vi "Main Page - Multi FPGA.vi"(8 "error in (no error)":errorcluster, 11 "Node Ptr":T1 format="%.0x") -> (0 "error out":errorcluster)   [LabVIEW 2015, in "Engine Simulation Toolkit System Explorer.lvlib"]
uses:
  Engine Simulation Toolkit System Explorer.lvlib
  <vilib>/NI Veristand/Custom Device API/Custom Device Item Ref.ctl
  Listbox State.ctl
  Shared/Properties.vi
  <vilib>/NI Veristand/Custom Device API/Get Item Property (I32).vi
  <vilib>/NI Veristand/Custom Device API/Get Item Property (String Array).vi
  <vilib>/NI Veristand/Custom Device API/Get Item Property (Dependent File).vi
  <vilib>/NI Veristand/Custom Device API/Get Item Property (String).vi
  <vilib>/NI Veristand/Custom Device API/Set Item Property (I32).vi
  Shared/Constants and GUIDs.vi
  <vilib>/NI Veristand/Custom Device API/Set Item Property (String Array).vi
  <vilib>/NI Veristand/Custom Device API/Set Item Property (String).vi
  <userlib>/_OpenG.lib/array/array.llb/Delete Elements from 2D Array (String)__ogtk.vi
  <vilib>/NI Veristand/Custom Device API/Custom Device API.lvlib
  Shared/Engine Simulation Toolkit Shared.lvlib
  <vilib>/NI Veristand/Custom Device Tools/Custom Device Utility Library/Custom Device Utility Library.lvlib
panel:
  in  "Reload bitfile":bool
  in  "Set master":bool
  in  "Remove bitfile":bool
  in  "Add bitfile":bool
  in  "Bitfile listbox":i32[](listbox) caption="Available APUs"
  in  "Header 3":cluster{"Section Name":string}={"Section Name"="Bitfile Selection"}
  in  "Remove APU":bool
  in  "Add APU":bool
  in  "APU listbox":i32[](listbox) caption="Available APUs"
  in  "Header 2":cluster{"Section Name":string}={"Section Name"="Available APUs"}
  in  "CPU":i32=-2
  in  "Rate decimation":i32=1 min=1
  in  "Execution priority":enum16{"Low", "Medium", "High"}(ring)=enum."Medium"
  out "CD Version":string caption="Custom device version"
  in  "Header":cluster{"Section Name":string}={"Section Name"="Engine Simulation Toolkit Settings"}
  in  "Name":string
  # "(-2: automatic)"
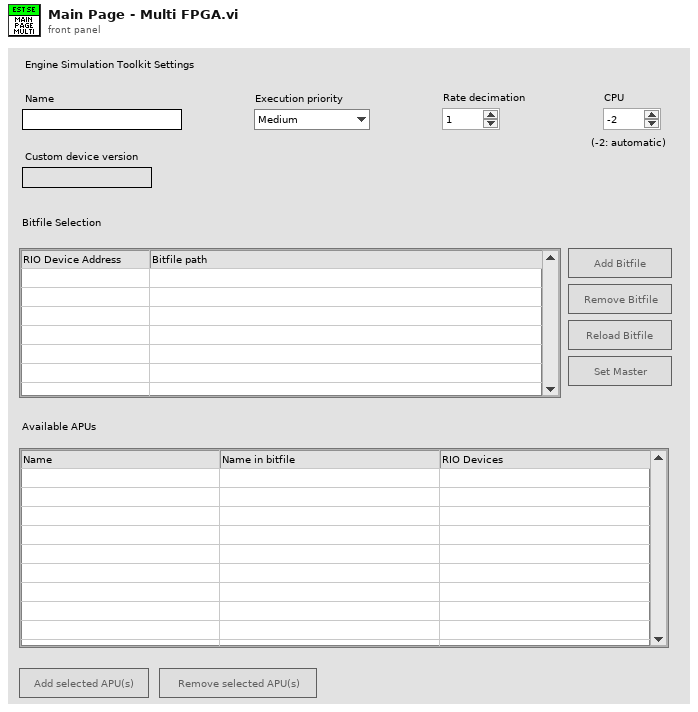
[diagram p1: front panel]
types:
  T1 = typedef "Custom Device API.lvlib/Custom Device Item Ref.ctl" = u64
  T2 = typedef "Engine Simulation Toolkit System Explorer.lvlib/Listbox State.ctl" = cluster{"listbox text":string[][], "not present item indexes":i32[], "selected values":i32[]}
  T3 = enum8{"Enabled", "Disabled", "Disabled and Grayed Out"}
  T4 = typedef "Custom Device API.lvlib/Custom Device Timed Loop Priority.ctl" = enum32{"Low", "Medium", "High"}
  T5 = typedef "Custom Device API.lvlib/Custom Device Item Info.ctl" = cluster{"Name":string, "Is Channel":bool, "GUID":string, "Is Waveform":bool}
  T6 = typedef "Custom Device API.lvlib/Custom Device Commands.ctl" = enum16{"Default", "Item renamed", "Shutdown", "Dynamic button pressed"}
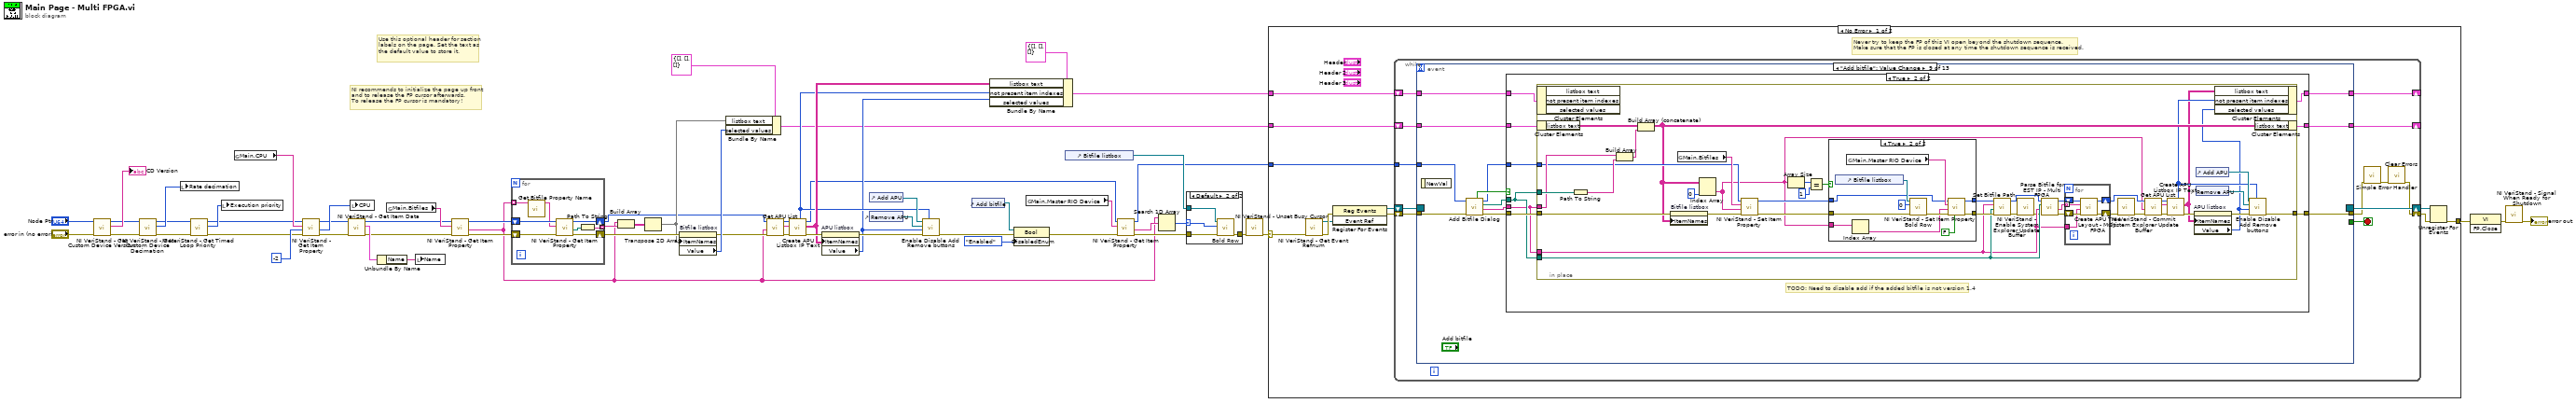
[diagram p0: block diagram]
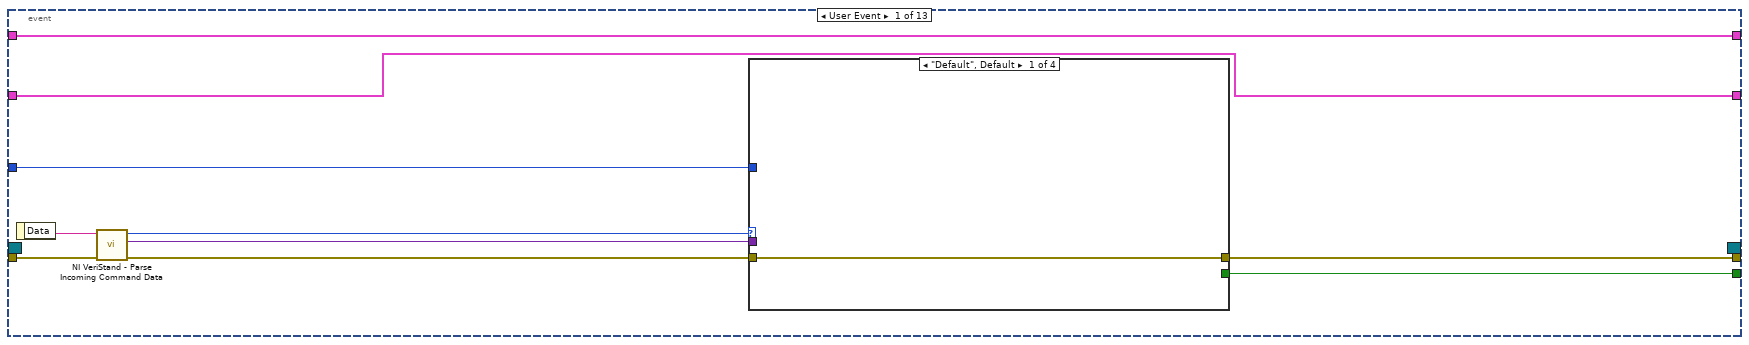
[diagram p3: hidden frame]
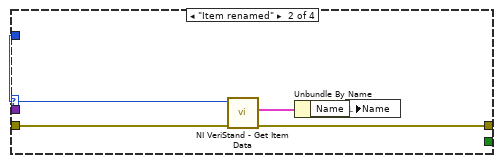
[diagram p4: hidden frame]
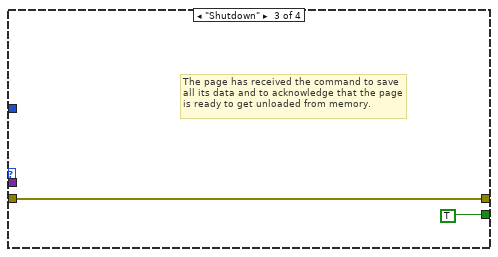
[diagram p5: hidden frame]
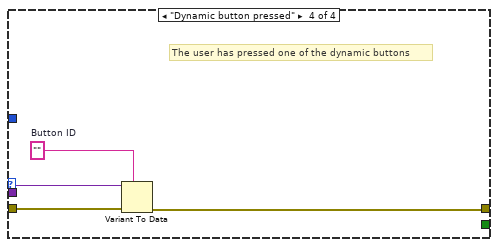
[diagram p6: hidden frame]
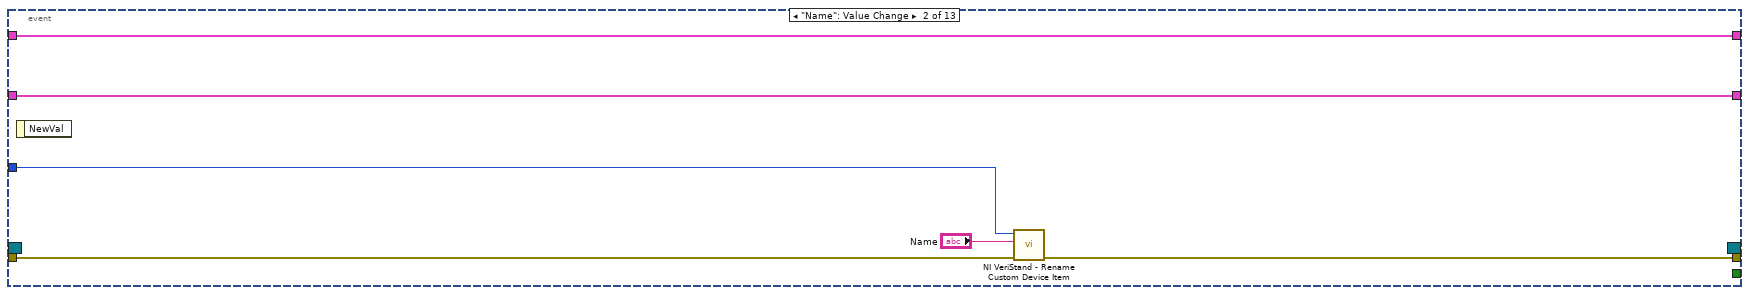
[diagram p7: hidden frame]
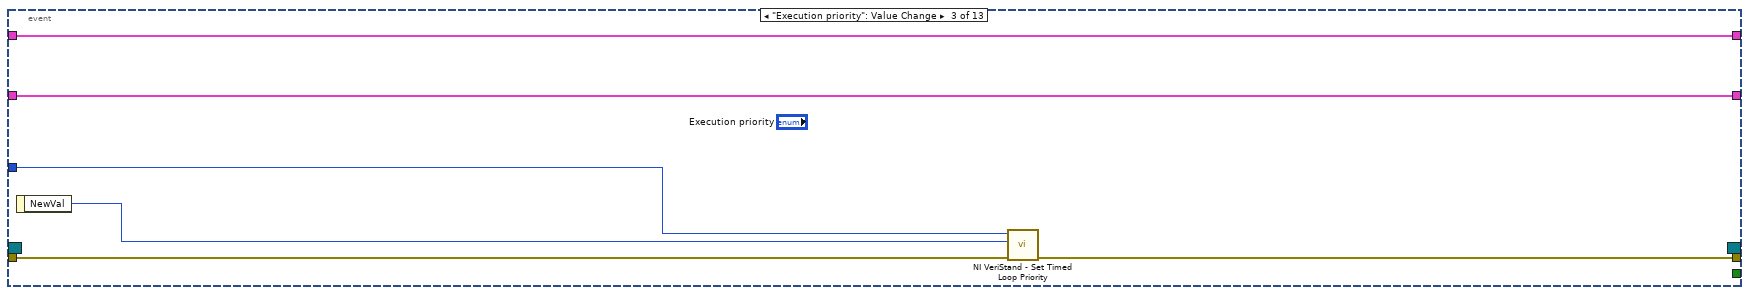
[diagram p8: hidden frame]
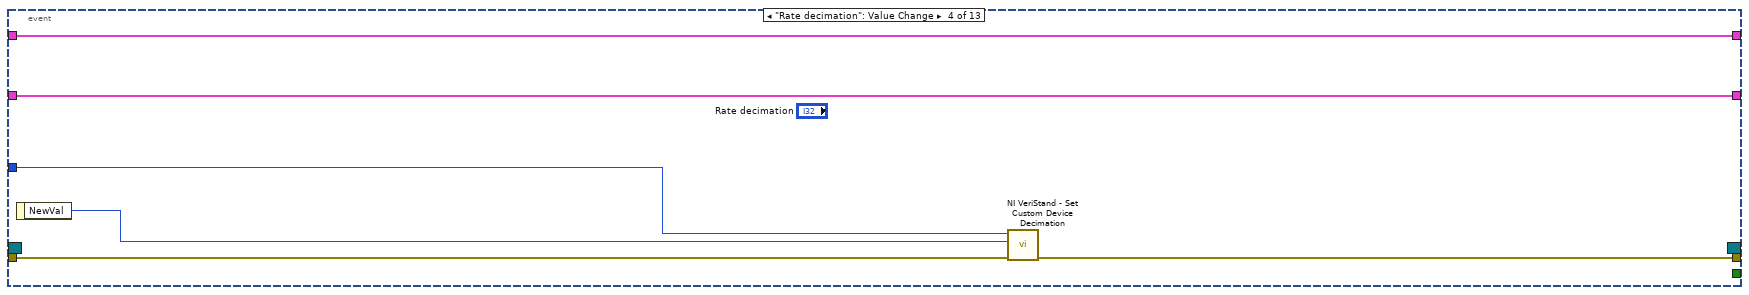
[diagram p9: hidden frame]
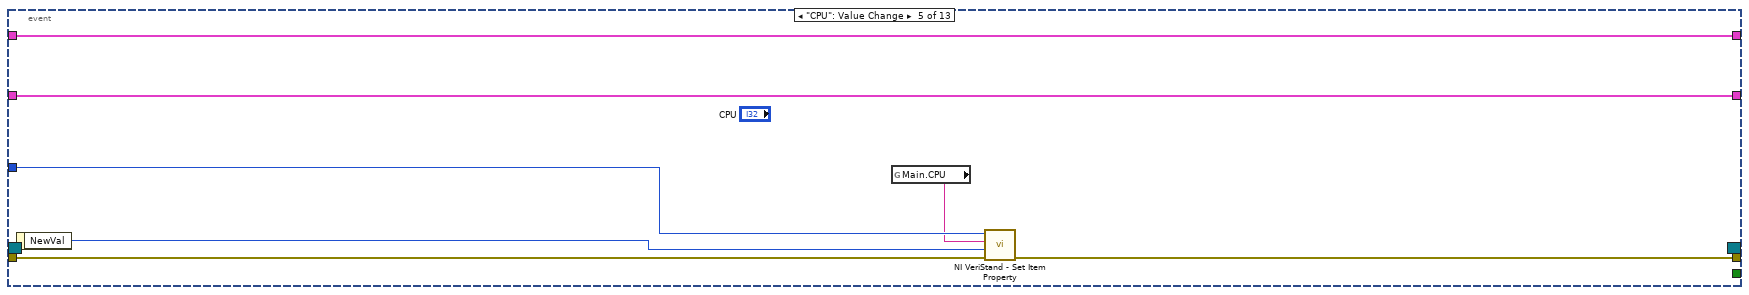
[diagram p10: hidden frame]
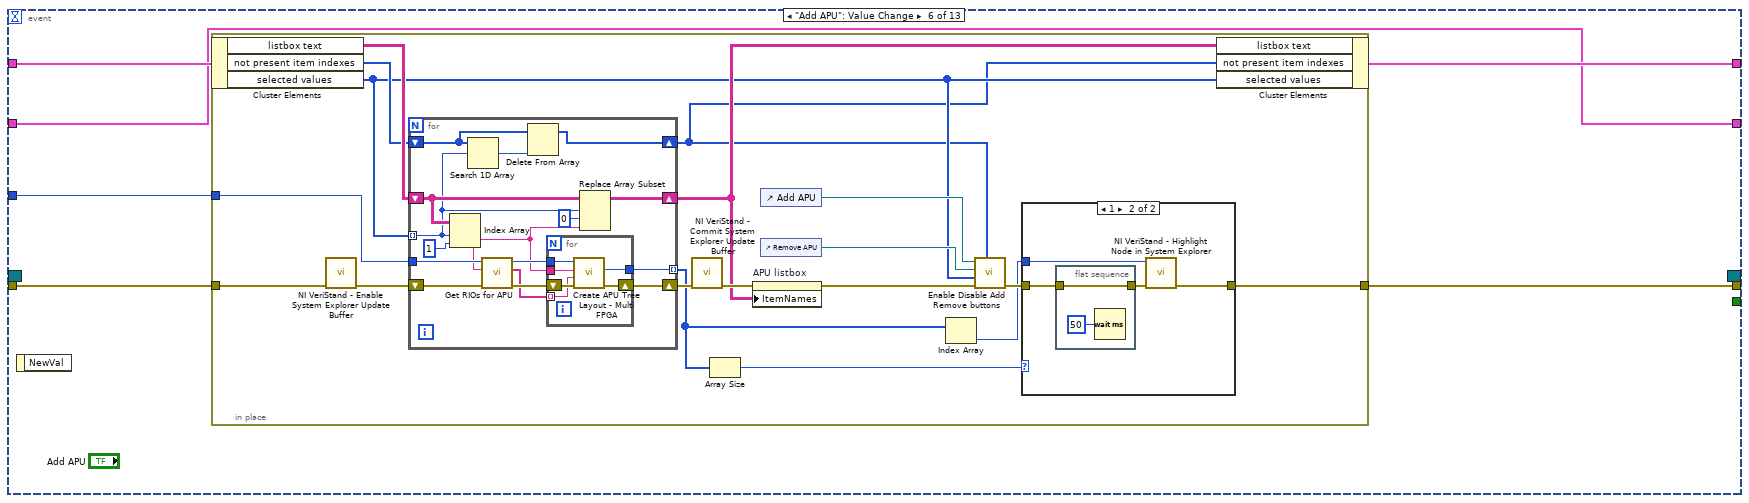
[diagram p11: hidden frame]
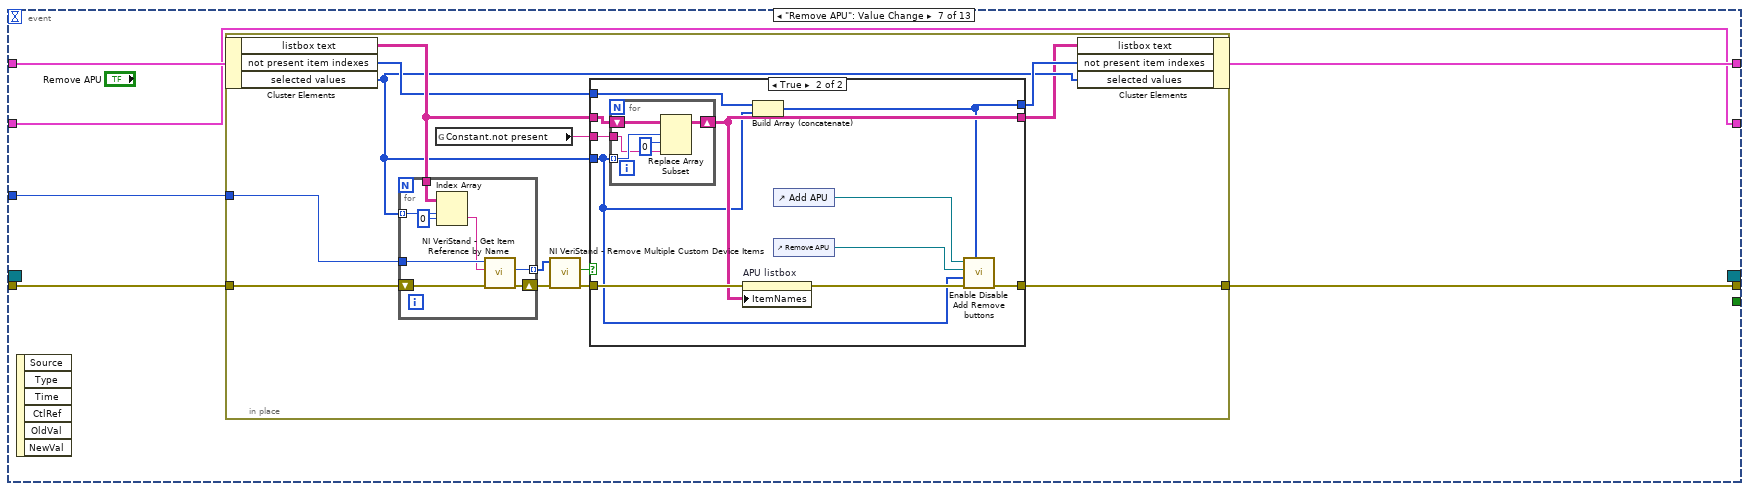
[diagram p13: hidden frame]
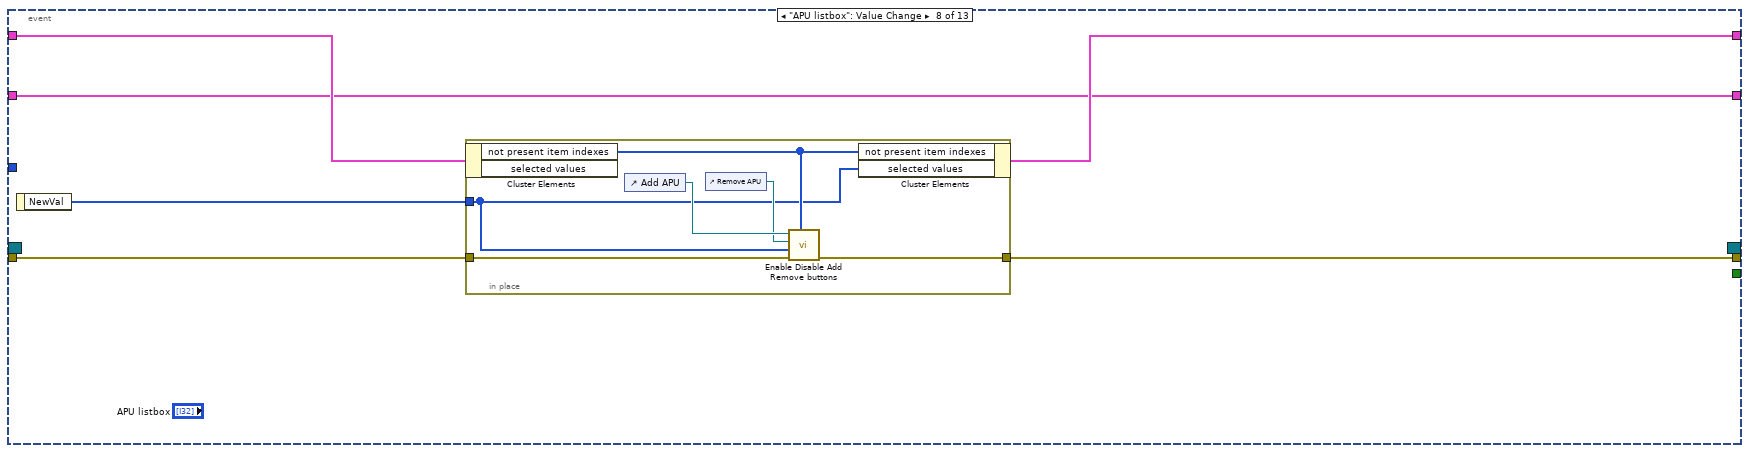
[diagram p15: hidden frame]
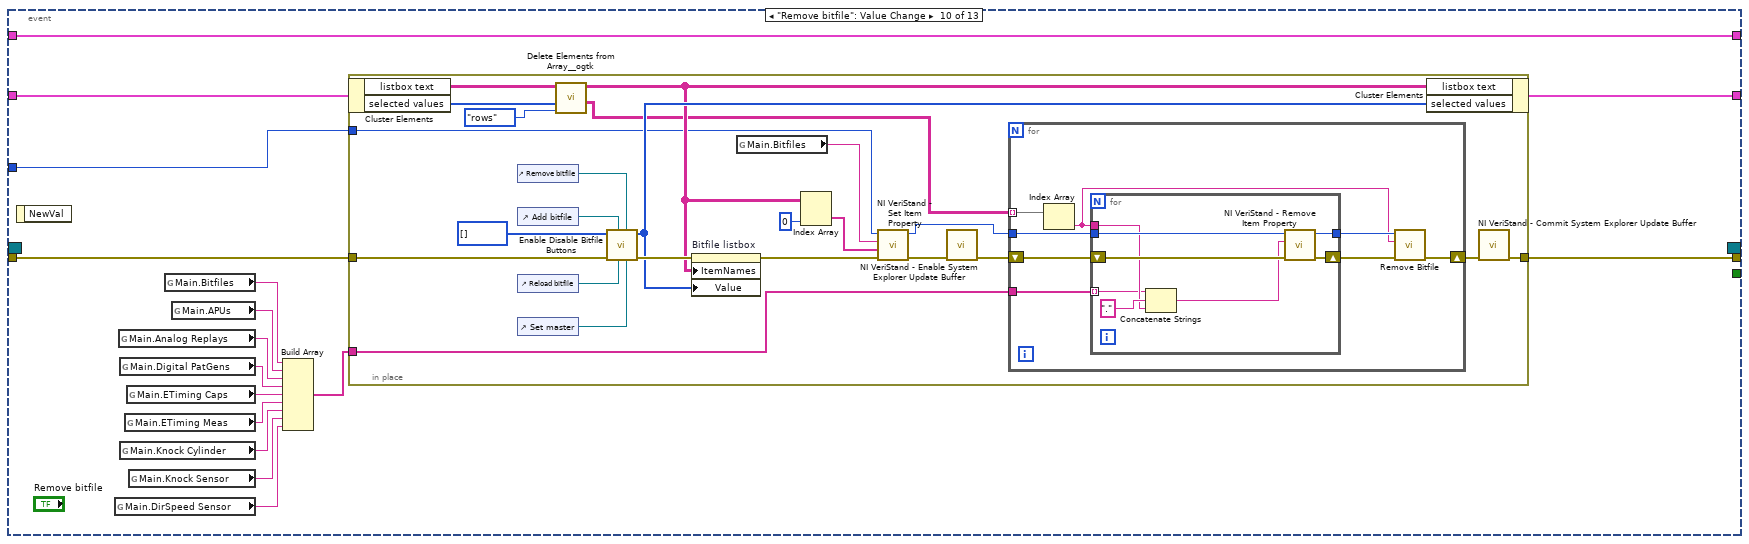
[diagram p18: hidden frame]
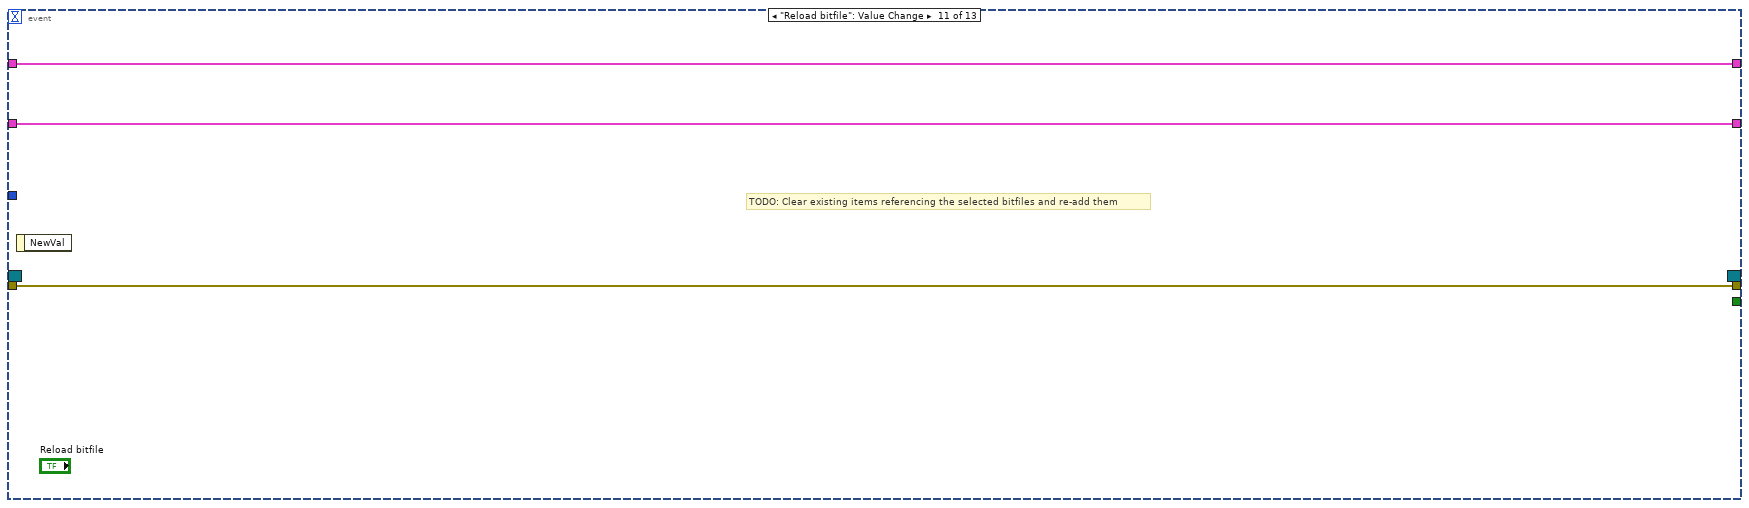
[diagram p19: hidden frame]
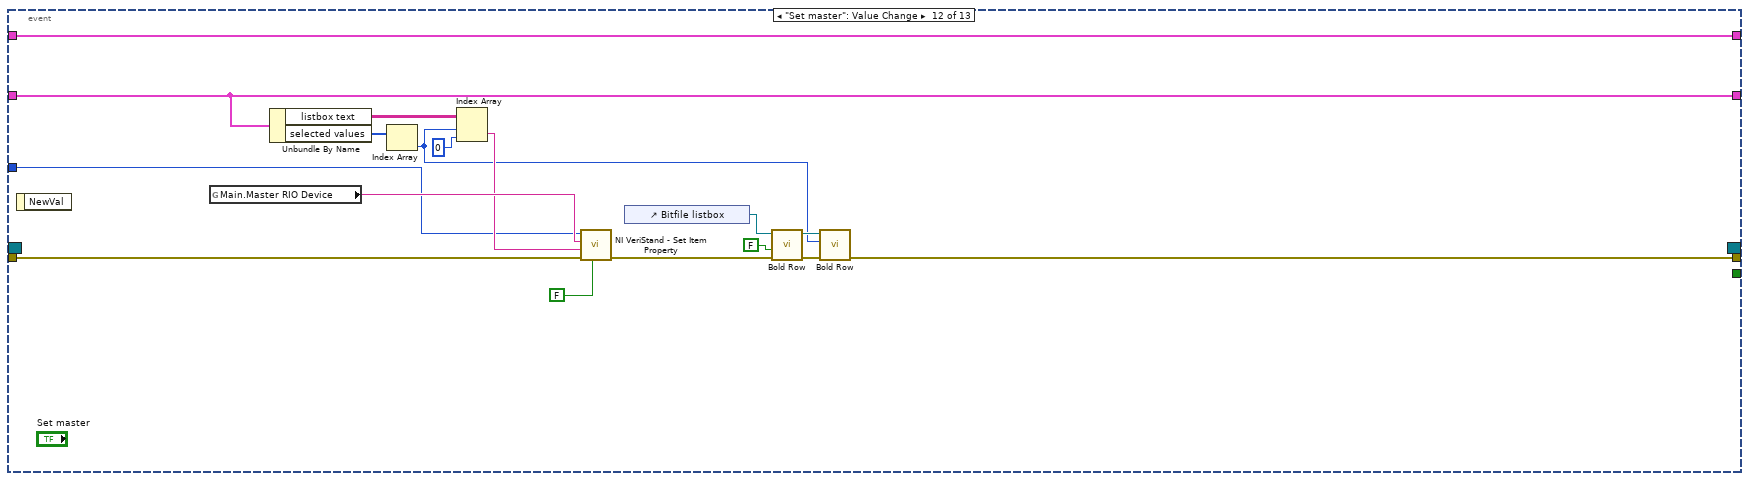
[diagram p20: hidden frame]
diagram:
  # "Use this optional header for section labels on the page. Set the text as the default value to store it."
  # "NI recommends to initialize the page up front\nand to release the FP cursor afterwards.\nTo release the FP cursor is mandatory!"
  n1 = call <vilib>:"NI VeriStand - Get Custom Device Version.vi"("error in (no error)"="error in (no error)", "Device Ref in"="Node Ptr") -> ("error out"=w54:errorcluster, "Value"=→"CD Version":string, "Device Ref out"=w51:T1)  [unwired: 7 in]
  n2 = call <vilib>:"NI VeriStand - Get Custom Device Decimation.vi"("error in (no error)"=w54, "Device Ref in"=w51) -> ("error out"=w52:errorcluster, "Decimation"=w50:i32, "Device Ref out"=w49:T1)  [unwired: 7 in]
  n3 = local write "Rate decimation"(w50) -> ()
  n4 = call <vilib>:"NI VeriStand - Get Timed Loop Priority.vi"("error in (no error)"=w52, "Device Ref in"=w49) -> ("error out"=w1:errorcluster, "Priority"=w48:T4, "Device Ref out"=w2:T1)  [unwired: 7 in]
  n5 = local write "Execution priority"(w48) -> ()
  n6 = global read "Properties.vi" "Main.CPU"() -> (w46:string)
  n7 = call-poly <vilib>:"NI VeriStand - Get Item Property.vi"("error in (no error)"=w1, "Default Value"=-2, "Property Name"=w46, "Item Ref in"=w2) -> ("error out"=w4:errorcluster, "Value"=w44:i32, "Item Ref out"=w5:T1)  [unwired: 4 in, 1 out]
  n8 = call <vilib>:"NI VeriStand - Get Item Data.vi"("error in (no error)"=w4, "Item Ref in"=w5) -> ("error out"=w11:errorcluster, "Item Info"=w56:T5, "Item Ref out"=w12:T1)  [unwired: 7 out]
  n9 = local write "CPU"(w44) -> ()
  n10 = Unbundle By Name(w56) -> ("Name"=w55:string)
  n11 = global read "Properties.vi" "Main.Bitfiles"() -> (w26:string)
  n12 = local write "Name"(w55) -> ()
  n13 = call-poly <vilib>:"NI VeriStand - Get Item Property.vi"("error in (no error)"=w11, "Property Name"=w26, "Item Ref in"=w12) -> ("error out"=w25:errorcluster, "Value"=w3:string[], "Item Ref out"=w23:T1)  [unwired: 5 in, 1 out]
  n14 = for {
    shift-right: [w68] -> w24
    shift-left: w25 -> [w69]
    tunnel: [w64] -> w22 mode=indexing
    shift-right: [w66] -> w8
    shift-left: w23 -> [w67]
    tunnel: w3 -> [w62] mode=indexing
    n15 = call "Get Bitfile Property Name.vi"("RIO Device Address in"=w62) -> ("Bitfile Property Name"=w63:string)  [unwired: 10 in]
    n16 = call-poly <vilib>:"NI VeriStand - Get Item Property.vi"("error in (no error)"=w69, "Property Name"=w63, "Item Ref in"=w67) -> ("error out"=w68:errorcluster, "Path"=w65:path, "Item Ref out"=w66:T1)  [unwired: 4 in, 2 out]
    n17 = Path To String(path=w65) -> (string=w64:string)
  }
  n18 = Build Array(w3, w22) -> (w21:string[][])
  n19 = Transpose 2D Array(2D array=w21) -> (transposed array=w20:string[][])
  n20 = property on="Bitfile listbox" class="MCListbox (strict)"(error in=w24, "ItemNames"=w20) -> (error out=w10:errorcluster, "Value"=w28:i32[])  [unwired: 1 in, 1 out]
  n21 = Bundle By Name(cluster=T2 {"listbox text"=[], "not present item indexes"=[], "selected values"=[]} ("output cluster"), "listbox text"=w20, "selected values"=w28) -> (w27:T2)
  n22 = call "Get APU List.vi"("error in (no error)"=w10, "rio names"=w3, "Item Ref in"=w8) -> ("error out"=w43:errorcluster, "ips available"=w41:string[], "Item Ref out"=w42:T1)  [unwired: 6 in]
  n23 = call "Create APU Listbox IP Text.vi"("error in (no error)"=w43, "ips available"=w41, "Section Ref in"=w42) -> ("error out"=w40:errorcluster, "listbox text"=w33:string[][], "Section Ref out"=w7:T1, "not present item indexes"=w32:i32[])  [unwired: 5 in]
  n24 = property on="APU listbox" class="MCListbox (strict)"(error in=w40, "ItemNames"=w33) -> (error out=w37:errorcluster, "Value"=w31:i32[])  [unwired: 1 in, 1 out]
  n25 = control-ref of="Add APU"() -> (w38:refnum<vi>)
  n26 = control-ref of="Remove APU"() -> (w39:refnum<vi>)
  n27 = call "Enable Disable Add Remove buttons.vi"("not present item indexes"=w32, "error in (no error)"=w37, "selected items"=w31, "remove button"=w39, "add button"=w38) -> ("error out"=w35:errorcluster)  [unwired: 6 in]
  n28 = control-ref of="Add bitfile"() -> (w36:refnum<vi>)
  n29 = Bundle By Name(cluster=T2 {"listbox text"=[], "not present item indexes"=[], "selected values"=[]} ("output cluster"), "listbox text"=w33, "not present item indexes"=w32, "selected values"=w31) -> (w30:T2)
  n30 = property on="Property Node" class="Bool"(reference=w36, error in=w35, "DisabledEnum"=T3."Enabled" ("Disabled")) -> (error out=w9:errorcluster)  [unwired: 1 out]
  n31 = global read "Properties.vi" "Main.Master RIO Device"() -> (w15:string)
  n32 = control-ref of="Bitfile listbox"() -> (w19:refnum<vi>)
  n33 = call-poly <vilib>:"NI VeriStand - Get Item Property.vi"("error in (no error)"=w9, "Property Name"=w15, "Item Ref in"=w7) -> ("error out"=w17:errorcluster, "Value"=w14:string, "Item Ref out"=w16:T1)  [unwired: 5 in, 1 out]
  n34 = Search 1D Array(1D array=w3, element=w14) -> (index of element=w13:i32)  [unwired: 1 in]
  n35 = case shown="Default" w13 {
    selector: w13 -> [_ w71]
    tunnel: w19 -> [_ w74]
    tunnel: [w70 w73] -> w18
    tunnel: w17 -> [w70 w72]
    frame -1 {
    }
    frame Default {
      n36 = call "Bold Row.vi"("error in (no error)"=w72, "Row (-2 : all)"=w71, "MulticolumnListbox in"=w74) -> ("error out"=w73:errorcluster)  [unwired: 7 in, 1 out]
    }
  }
  n37 = call <vilib>:"NI VeriStand - Unset Busy Cursor.vi"("error in (no error)"=w18) -> ("error out"=w58:errorcluster)  [unwired: 10 out]
  n38 = case shown="No Error" w58 {
    selector: w58 -> [w77 w429]
    tunnel: [w82 w427] -> w61
    tunnel: w16 -> [w78 _]
    tunnel: w30 -> [w76 _]
    tunnel: w27 -> [w75 _]
    frame No Error {
      # "Never try to keep the FP of this VI open beyond the shutdown sequence.\nMake sure that the FP is closed at any time the shutdown sequence is received."
      n39 = call <vilib>:"NI VeriStand - Get Event Refnum.vi"("error in (no error)"=w77) -> ("error out"=w85:errorcluster, "Event Ref"=w81:refnum<user-event>)  [unwired: 9 out]
      n40 = register-events(error in=w85, w81) -> (reference out=w79:refnum<event-registration>, error out=w80:errorcluster)  [unwired: 1 in]
      n41 = while {
        tunnel: w78 -> [w93]
        shift-right: [w90] -> w83
        shift-left: w80 -> [w96]
        shift-right: [w97] -> w84
        shift-left: w79 -> [w95]
        shift-right: [w88] -> _
        shift-left: w76 -> [w89]
        shift-right: [w86] -> _
        shift-left: w75 -> [w87]
        stop <- w94 stop-if-true
        n42 = event shown="[8] \"Add bitfile\": Value Change" {
          selector: w95 -> [_ _ _ _ _ _ _ _ _ _ _ _ _]
          dyn-events: [_ _ _ _ _ _ _ _ _ _ _ _ _] -> w97
          timeout: _ -> [_ _ _ _ _ _ _ _ _ _ _ _ _]
          tunnel: w96 -> [w107 w125 w131 w137 w144 w150 w203 w249 w264 w355 w398 w407 w426]
          tunnel: [w103 _ _ _ _ _ _ _ _ _ _ _ _] -> w94
          tunnel: [w102 w124 w129 w135 w140 w149 w202 w248 w267 w340 w398 w403 w424] -> w92
          tunnel: w93 -> [w101 w123 w130 w136 w143 w148 w201 _ w259 w351 _ w408 _]
          tunnel: w89 -> [w99 w121 w127 w133 w139 w147 w200 w246 w257 w352 w397 w415 w419]
          tunnel: [w99 w121 w127 w133 w139 w146 w199 w245 w256 w352 w397 w415 w419] -> w88
          tunnel: w87 -> [w98 w120 w126 w132 w138 w145 w198 w244 w266 w354 w396 w414 w418]
          tunnel: [w98 w120 w126 w132 w138 w145 w198 w244 w265 w353 w396 w414 w417] -> w86
          event User Event {
            n43 = event-data() -> ("Data"=w106:string)  [unwired: 1 out]
            n44 = call <vilib>:"NI VeriStand - Parse Incoming Command Data.vi"("error in (no error)"=w107, "Incoming data"=w106) -> ("error out"=w105:errorcluster, "Outgoing data"=w100:variant, "Action"=w104:T6)  [unwired: 7 out]
            n45 = case shown="\"Default\", Default" w104 {
              tunnel: w105 -> [w108 w113 w114 w119]
              tunnel: [_ _ TRUE _] -> w103
              tunnel: [w108 w110 w114 w116] -> w102
              tunnel: w101 -> [_ w112 _ _]
              tunnel: w100 -> [_ _ _ w118]
              frame "Default", Default {
              }
              frame "Item renamed" {
                n46 = call <vilib>:"NI VeriStand - Get Item Data.vi"("error in (no error)"=w113, "Item Ref in"=w112) -> ("error out"=w110:errorcluster, "Item Info"=w111:T5)  [unwired: 8 out]
                n47 = Unbundle By Name(w111) -> ("Name"=w109:string)
                n48 = local write "Name"(w109) -> ()
              }
              frame "Shutdown" {
                # "The page has received the command to save all its data and to acknowledge that the page is ready to get unloaded from memory."
              }
              frame "Dynamic button pressed" {
                w117 = ""  # Button ID
                # "The user has pressed one of the dynamic buttons"
                n49 = Variant To Data(error in=w119, type=w117, Variant=w118) -> (error out=w116:errorcluster)  [unwired: 1 out]
              }
            }
          }
          event "Name": Value Change {
            n50 = event-data() -> ()  [unwired: 2 out]
            n51 = call <vilib>:"NI VeriStand - Rename Custom Device Item.vi"("error in (no error)"=w125, "New Name"="Name", "Item Ref in"=w123) -> ("error out"=w124:errorcluster)  [unwired: 1 in, 7 out]
          }
          event "Execution priority": Value Change {
            n52 = event-data() -> ("NewVal"=w128:enum16{"Low", "Medium", "High"})  [unwired: 1 out]
            n53 = call <vilib>:"NI VeriStand - Set Timed Loop Priority.vi"("error in (no error)"=w131, "Priority"=w128, "Device Ref in"=w130) -> ("error out"=w129:errorcluster)  [unwired: 7 in, 1 out]
          }
          event "Rate decimation": Value Change {
            n54 = event-data() -> ("NewVal"=w134:i32)  [unwired: 1 out]
            n55 = call <vilib>:"NI VeriStand - Set Custom Device Decimation.vi"("error in (no error)"=w137, "Decimation"=w134, "Device Ref in"=w136) -> ("error out"=w135:errorcluster)  [unwired: 7 in, 1 out]
          }
          event "CPU": Value Change {
            n56 = event-data() -> ("NewVal"=w142:i32)  [unwired: 1 out]
            n57 = global read "Properties.vi" "Main.CPU"() -> (w141:string)
            n58 = call-poly <vilib>:"NI VeriStand - Set Item Property.vi"("error in (no error)"=w144, "Value"=w142, "Property Name"=w141, "Item Ref in"=w143) -> ("error out"=w140:errorcluster)  [unwired: 5 in, 2 out]
          }
          event "Add APU": Value Change {
            n59 = event-data() -> ()  [unwired: 2 out]
            n60 = in-place {
              in-place-border: w150 -> [w158]
              in-place-border: [w157] -> w149
              in-place-border: w148 -> [w156]
              n61 = in-place-cluster #1(w147) -> ("listbox text"=w155:string[][], "not present item indexes"=w154:i32[], "selected values"=w152:i32[])
              n62 = call <vilib>:"NI VeriStand - Enable System Explorer Update Buffer.vi"("error in (no error)"=w158) -> ("error out"=w163:errorcluster)  [unwired: 10 in]
              n63 = for {
                tunnel: w156 -> [w179]
                shift-right: [w191] -> w168
                shift-left: w163 -> [w178]
                tunnel: w152 -> [w186] mode=indexing
                shift-right: [w188] -> w153
                shift-left: w155 -> [w189]
                shift-right: [w183] -> w151
                shift-left: w154 -> [w185]
                tunnel: [w182] -> w161 mode=indexing
                n64 = Index Array(array=w189, index (row)=w186, index (col)=1 ("disabled index (col)")) -> (element=w176:string)
                n65 = Search 1D Array(1D array=w185, element=w186) -> (index of element=w184:i32)  [unwired: 1 in]
                n66 = call "Get RIOs for APU.vi"("error in (no error)"=w178, "APU name"=w176, "Item Ref in"=w179) -> ("error out"=w181:errorcluster, "RIO Addresses"=w177:string[], "Item Ref out"=w180:T1)  [unwired: 6 in]
                n67 = Delete From Array(array=w185, index=w184) -> (array with subset deleted=w183:i32[])  [unwired: 1 in, 1 out]
                n68 = for {
                  tunnel: w176 -> [w196]
                  shift-right: [w197] -> w191
                  shift-left: w181 -> [w194]
                  tunnel: w177 -> [w192] mode=indexing
                  tunnel: w180 -> [w193]
                  tunnel: [w195] -> w182
                  n69 = call "Create APU Tree Layout - Multi FPGA.vi"("error in (no error)"=w194, "rio name"=w192, "engine name"=w196, "Section Ptr"=w193) -> ("error out"=w197:errorcluster, "APU ref"=w195:T1)  [unwired: 5 in, 1 out]
                }
                n70 = Replace Array Subset(array=w189, new element=w176, index (row)=w186, index (col)=0 ("disabled index (col)")) -> (w188:string[][])
              }
              n71 = call <vilib>:"NI VeriStand - Commit System Explorer Update Buffer.vi"("error in (no error)"=w168) -> ("error out"=w162:errorcluster)  [unwired: 10 in]
              n72 = Array Size(array=w161) -> (size(s)=w159:i32)
              n73 = property on="APU listbox" class="MCListbox (strict)"(error in=w162, "ItemNames"=w153) -> (error out=w167:errorcluster)  [unwired: 1 in, 1 out]
              n74 = control-ref of="Add APU"() -> (w165:refnum<vi>)
              n75 = control-ref of="Remove APU"() -> (w164:refnum<vi>)
              n76 = Index Array(array=w161) -> (element=w160:T1)  [unwired: 1 in]
              n77 = call "Enable Disable Add Remove buttons.vi"("not present item indexes"=w151, "error in (no error)"=w167, "selected items"=w152, "remove button"=w164, "add button"=w165) -> ("error out"=w166:errorcluster)  [unwired: 6 in]
              n78 = case shown="1" w159 {
                tunnel: w166 -> [w169 w170]
                tunnel: [w169 w173] -> w157
                tunnel: w160 -> [_ w172]
                frame Default {
                }
                frame 1 {
                  n79 = flat-sequence {
                    tunnel: [w174] -> w171
                    tunnel: w170 -> [w174]
                    frame #0 {
                      n80 = Wait (ms)(milliseconds to wait=u32 50) -> ()  [unwired: 1 out]
                    }
                  }
                  n81 = call <vilib>:"NI VeriStand - Highlight Node in System Explorer.vi"("error in (no error)"=w171, "Item Ref in"=w172) -> ("error out"=w173:errorcluster)  [unwired: 8 in, 1 out]
                }
              }
              n82 = in-place-cluster #1("listbox text"=w153, "not present item indexes"=w151, "selected values"=w152) -> (w146:T2)
            }
          }
          event "Remove APU": Value Change {
            n83 = event-data() -> ()  [unwired: 7 out]
            n84 = in-place {
              in-place-border: w203 -> [w211]
              in-place-border: [w210] -> w202
              in-place-border: w201 -> [w209]
              n85 = in-place-cluster #2(w200) -> ("listbox text"=w208:string[][], "not present item indexes"=w206:i32[], "selected values"=w205:i32[])
              n86 = for {
                tunnel: w205 -> [w242] mode=indexing
                tunnel: w208 -> [w243]
                tunnel: w209 -> [w239]
                tunnel: [w236] -> w215 mode=indexing
                shift-right: [w238] -> w216
                shift-left: w211 -> [w240]
                n87 = Index Array(array=w243, index (row)=w242, index (col)=0 ("disabled index (col)")) -> (element=w237:string)
                n88 = call <vilib>:"NI VeriStand - Get Item Reference by Name.vi"("error in (no error)"=w240, "Item Name"=w237, "Parent Ref in"=w239) -> ("error out"=w238:errorcluster, "Item Ref"=w236:T1)  [unwired: 5 in, 2 out]
              }
              n89 = global read "Constants and GUIDs.vi" "Constant.not present"() -> (w212:string)
              n90 = call <vilib>:"NI VeriStand - Remove Multiple Custom Device Items.vi"("error in (no error)"=w216, "Item Refs in"=w215) -> ("error out"=w214:errorcluster, "Deleted?"=w213:bool)  [unwired: 8 in]
              n91 = case shown="True" w213 {
                tunnel: [w218 w229] -> w210
                tunnel: w214 -> [w218 w226]
                tunnel: w205 -> [_ w221]
                tunnel: w208 -> [w219 w225]
                tunnel: w212 -> [_ w224]
                tunnel: [w219 w223] -> w204
                tunnel: w206 -> [w217 w222]
                tunnel: [w217 w220] -> w207
                frame False {
                }
                frame True {
                  n92 = for {
                    tunnel: w221 -> [w233] mode=indexing
                    shift-right: [w234] -> w223
                    shift-left: w225 -> [w235]
                    tunnel: w224 -> [w231]
                    n93 = Replace Array Subset(array=w235, new element=w231, index (row)=w233, index (col)=0 ("disabled index (col)")) -> (w234:string[][])
                  }
                  n94 = property on="APU listbox" class="MCListbox (strict)"(error in=w226, "ItemNames"=w223) -> (error out=w230:errorcluster)  [unwired: 1 in, 1 out]
                  n95 = Build Array (concatenate)(w222, w221) -> (w220:i32[])
                  n96 = control-ref of="Add APU"() -> (w228:refnum<vi>)
                  n97 = control-ref of="Remove APU"() -> (w227:refnum<vi>)
                  n98 = call "Enable Disable Add Remove buttons.vi"("not present item indexes"=w220, "error in (no error)"=w230, "selected items"=w221, "remove button"=w227, "add button"=w228) -> ("error out"=w229:errorcluster)  [unwired: 6 in]
                }
              }
              n99 = in-place-cluster #2("listbox text"=w204, "not present item indexes"=w207, "selected values"=w205) -> (w199:T2)
            }
          }
          event "APU listbox": Value Change {
            n100 = event-data() -> ("NewVal"=w247:i32[])  [unwired: 1 out]
            n101 = in-place {
              in-place-border: w249 -> [w253]
              in-place-border: [w252] -> w248
              in-place-border: w247 -> [w250]
              n102 = in-place-cluster #3(w246) -> ("not present item indexes"=w251:i32[])  [unwired: 1 out]
              n103 = control-ref of="Add APU"() -> (w255:refnum<vi>)
              n104 = control-ref of="Remove APU"() -> (w254:refnum<vi>)
              n105 = call "Enable Disable Add Remove buttons.vi"("not present item indexes"=w251, "error in (no error)"=w253, "selected items"=w250, "remove button"=w254, "add button"=w255) -> ("error out"=w252:errorcluster)  [unwired: 6 in]
              n106 = in-place-cluster #3("not present item indexes"=w251, "selected values"=w250) -> (w245:T2)
            }
          }
          event "Add bitfile": Value Change {
            n107 = event-data() -> ()  [unwired: 2 out]
            n108 = call "Add Bitfile Dialog.vi"("error in (no error)"=w264, "Item Ref in"=w259) -> ("error out"=w262:errorcluster, "RIO Device Address out"=w261:string, "Bitfile Path out"=w263:path, "Item Ref out"=w258:T1, "OK?"=w260:bool)  [unwired: 5 in]
            n109 = case shown="True" w260 {
              tunnel: w262 -> [w269 w279]
              tunnel: [w269 w275] -> w267
              tunnel: w266 -> [w270 w278]
              tunnel: [w270 w277] -> w265
              tunnel: w263 -> [_ w274]
              tunnel: w261 -> [_ w273]
              tunnel: w258 -> [_ w276]
              tunnel: w257 -> [w268 w272]
              tunnel: [w268 w271] -> w256
              frame False {
              }
              frame True {
                # "TODO: Need to disable add if the added bitfile is not version 1.4"
                n110 = in-place {
                  in-place-border: [w298] -> w275
                  in-place-border: w274 -> [w318]
                  in-place-border: w273 -> [w316]
                  in-place-border: w279 -> [w315]
                  in-place-border: w276 -> [w313]
                  in-place-border: w274 -> [w291]
                  in-place-border: w273 -> [w286]
                  n111 = in-place-cluster #4(w272) -> ()  [unwired: 3 out]
                  n112 = in-place-cluster #5(w278) -> ("listbox text"=w320:string[][])
                  n113 = Path To String(path=w318) -> (string=w317:string)
                  n114 = Build Array(w316, w317) -> (w319:string[])
                  n115 = Build Array (concatenate)(w320, w319) -> (w308:string[][])
                  n116 = property on="Bitfile listbox" class="MCListbox (strict)"(error in=w315, "ItemNames"=w308) -> (error out=w311:errorcluster)  [unwired: 1 in, 1 out]
                  n117 = global read "Properties.vi" "Main.Bitfiles"() -> (w314:string)
                  n118 = Index Array(array=w308, index (col)=0 ("disabled index (col)")) -> (element=w282:string[])  [unwired: 1 in]
                  n119 = call-poly <vilib>:"NI VeriStand - Set Item Property.vi"("error in (no error)"=w311, "Value"=w282, "Property Name"=w314, "Item Ref in"=w313) -> ("error out"=w310:errorcluster, "Item Ref out"=w309:T1)  [unwired: 5 in, 1 out]
                  n120 = Array Size(array=w282) -> (size(s)=w307:i32)
                  n121 = Equal?(x=w307, y=1) -> (x = y?=w305:bool)
                  n122 = case shown="True" w305 {
                    tunnel: [w327 w334] -> w294
                    tunnel: w310 -> [w327 w333]
                    tunnel: w309 -> [w328 w332]
                    tunnel: [w328 w331] -> w293
                    tunnel: w282 -> [_ w330]
                    frame False {
                    }
                    frame True {
                      n123 = control-ref of="Bitfile listbox"() -> (w339:refnum<vi>)
                      n124 = global read "Properties.vi" "Main.Master RIO Device"() -> (w337:string)
                      n125 = Index Array(array=w330) -> (element=w329:string)  [unwired: 1 in]
                      n126 = call "Bold Row.vi"("error in (no error)"=w333, "Row (-2 : all)"=0, "MulticolumnListbox in"=w339) -> ("error out"=w335:errorcluster)  [unwired: 7 in, 1 out]
                      n127 = call-poly <vilib>:"NI VeriStand - Set Item Property.vi"("Binary String (T)"=FALSE ("Binary String"), "error in (no error)"=w335, "Value"=w329, "Property Name"=w337, "Item Ref in"=w332) -> ("error out"=w334:errorcluster, "Item Ref out"=w331:T1)  [unwired: 4 in, 1 out]
                    }
                  }
                  n128 = call "Set Bitfile Path.vi"("error in (no error)"=w294, "Bitfile Path in"=w291, "RIO Device Address in"=w286, "Item Ref in"=w293) -> ("error out"=w296:errorcluster, "Item Ref out"=w297:T1)  [unwired: 6 in]
                  n129 = call <vilib>:"NI VeriStand - Enable System Explorer Update Buffer.vi"("error in (no error)"=w296) -> ("error out"=w281:errorcluster)  [unwired: 10 in]
                  n130 = call "Parse Bitfile for EST IP - Multi FPGA.vi"("error in (no error)"=w281, "RIO device address"=w286, "bitfile path"=w291, "Item Ref in"=w297) -> ("error out"=w287:errorcluster, "APUs"=w285:string[], "Item Ref out"=w283:T1)  [unwired: 4 in, 1 out]
                  n131 = for {
                    shift-right: [w325] -> w295
                    shift-left: w287 -> [w326]
                    tunnel: w285 -> [w323] mode=indexing
                    tunnel: w286 -> [w322]
                    shift-right: [w321] -> w292
                    shift-left: w283 -> [w324]
                    n132 = call "Create APU Tree Layout - Multi FPGA.vi"("error in (no error)"=w326, "rio name"=w322, "engine name"=w323, "Section Ptr"=w324) -> ("error out"=w325:errorcluster, "Section Ptr dup"=w321:T1)  [unwired: 5 in, 1 out]
                  }
                  n133 = call <vilib>:"NI VeriStand - Commit System Explorer Update Buffer.vi"("error in (no error)"=w295) -> ("error out"=w280:errorcluster)  [unwired: 10 in]
                  n134 = call "Get APU List.vi"("error in (no error)"=w280, "rio names"=w282, "Item Ref in"=w292) -> ("error out"=w304:errorcluster, "ips available"=w284:string[], "Item Ref out"=w303:T1)  [unwired: 6 in]
                  n135 = call "Create APU Listbox IP Text.vi"("error in (no error)"=w304, "ips available"=w284, "Section Ref in"=w303) -> ("error out"=w299:errorcluster, "listbox text"=w289:string[][], "not present item indexes"=w290:i32[])  [unwired: 5 in, 1 out]
                  n136 = property on="APU listbox" class="MCListbox (strict)"(error in=w299, "ItemNames"=w289) -> (error out=w302:errorcluster, "Value"=w288:i32[])  [unwired: 1 in, 1 out]
                  n137 = control-ref of="Add APU"() -> (w300:refnum<vi>)
                  n138 = control-ref of="Remove APU"() -> (w301:refnum<vi>)
                  n139 = in-place-cluster #4("listbox text"=w289, "not present item indexes"=w290, "selected values"=w288) -> (w271:T2)
                  n140 = call "Enable Disable Add Remove buttons.vi"("not present item indexes"=w290, "error in (no error)"=w302, "selected items"=w288, "remove button"=w301, "add button"=w300) -> ("error out"=w298:errorcluster)  [unwired: 6 in]
                  n141 = in-place-cluster #5("listbox text"=w308) -> (w277:T2)
                }
              }
            }
          }
          event "Remove bitfile": Value Change {
            n142 = event-data() -> ()  [unwired: 2 out]
            n143 = global read "Properties.vi" "Main.DirSpeed Sensor"() -> (w343:string)
            n144 = global read "Properties.vi" "Main.Analog Replays"() -> (w350:string)
            n145 = global read "Properties.vi" "Main.Digital PatGens"() -> (w349:string)
            n146 = global read "Properties.vi" "Main.Knock Cylinder"() -> (w345:string)
            n147 = global read "Properties.vi" "Main.ETiming Meas"() -> (w347:string)
            n148 = global read "Properties.vi" "Main.ETiming Caps"() -> (w348:string)
            n149 = global read "Properties.vi" "Main.Knock Sensor"() -> (w344:string)
            n150 = global read "Properties.vi" "Main.Bitfiles"() -> (w342:string)
            n151 = global read "Properties.vi" "Main.APUs"() -> (w346:string)
            n152 = Build Array(w342, w346, w350, w349, w348, w347, w345, w344, w343) -> (w341:string[])
            n153 = in-place {
              in-place-border: w355 -> [w372]
              in-place-border: [w356] -> w340
              in-place-border: w351 -> [w361]
              in-place-border: w341 -> [w359]
              n154 = in-place-cluster #6(w354) -> ("listbox text"=w379:string[][], "selected values"=w378:i32[])
              n155 = control-ref of="Remove bitfile"() -> (w375:refnum<vi>)
              n156 = control-ref of="Add bitfile"() -> (w376:refnum<vi>)
              n157 = control-ref of="Reload bitfile"() -> (w374:refnum<vi>)
              n158 = control-ref of="Set master"() -> (w373:refnum<vi>)
              n159 = call-poly <userlib>:"Delete Elements from Array__ogtk.vi"("delete (rows or columns)"=enum16{"rows", "columns"}."rows", "indices"=w378, "array"=w379) -> ("deleted elements"=w360:string[][], "array w/ subset deleted"=w366:string[][])  [unwired: 7 in]
              n160 = call "Enable Disable Bitfile Buttons.vi"("Set Master in"=w373, "Remove in"=w375, "Reload in"=w374, "Add in"=w376, "error in (no error)"=w372, "NewVal"=i32[] [] ("selected values")) -> ("error out"=w370:errorcluster, "NewVal"=w369:i32[])  [unwired: 4 in]
              n161 = property on="Bitfile listbox" class="MCListbox (strict)"(error in=w370, "ItemNames"=w366, "Value"=w369) -> (error out=w364:errorcluster)  [unwired: 1 in, 1 out]
              n162 = global read "Properties.vi" "Main.Bitfiles"() -> (w365:string)
              n163 = Index Array(array=w366, index (col)=0 ("disabled index (col)")) -> (element=w368:string[])  [unwired: 1 in]
              n164 = call-poly <vilib>:"NI VeriStand - Set Item Property.vi"("error in (no error)"=w364, "Value"=w368, "Property Name"=w365, "Item Ref in"=w361) -> ("error out"=w363:errorcluster, "Item Ref out"=w362:T1)  [unwired: 5 in, 1 out]
              n165 = call <vilib>:"NI VeriStand - Enable System Explorer Update Buffer.vi"("error in (no error)"=w363) -> ("error out"=w357:errorcluster)  [unwired: 10 in]
              n166 = for {
                tunnel: w362 -> [w386]
                shift-right: [w381] -> w358
                shift-left: w357 -> [w387]
                tunnel: w360 -> [w385] mode=indexing
                tunnel: w359 -> [w384]
                n167 = Index Array(array=w385) -> (element=w380:string)  [unwired: 1 in]
                n168 = for {
                  tunnel: w386 -> [w394]
                  tunnel: w380 -> [w391]
                  shift-right: [w393] -> w383
                  shift-left: w387 -> [w395]
                  tunnel: w384 -> [w390] mode=indexing
                  tunnel: [w388] -> w382
                  n169 = Concatenate Strings(w390, "." ("string"), w391) -> (w389:string)
                  n170 = call <vilib>:"NI VeriStand - Remove Item Property.vi"("error in (no error)"=w395, "Property Name"=w389, "Item Ref in"=w394) -> ("error out"=w393:errorcluster, "Item Ref out"=w388:T1)  [unwired: 6 in, 1 out]
                }
                n171 = call "Remove Bitfile.vi"("error in (no error)"=w383, "RIO name"=w380, "Item Ref in"=w382) -> ("error out"=w381:errorcluster)  [unwired: 7 in, 1 out]
              }
              n172 = in-place-cluster #6("listbox text"=w366, "selected values"=w369) -> (w353:T2)
              n173 = call <vilib>:"NI VeriStand - Commit System Explorer Update Buffer.vi"("error in (no error)"=w358) -> ("error out"=w356:errorcluster)  [unwired: 10 in]
            }
          }
          event "Reload bitfile": Value Change {
            # "TODO: Clear existing items referencing the selected bitfiles and re-add them"
            n174 = event-data() -> ()  [unwired: 2 out]
          }
          event "Set master": Value Change {
            n175 = event-data() -> ()  [unwired: 2 out]
            n176 = global read "Properties.vi" "Main.Master RIO Device"() -> (w410:string)
            n177 = Unbundle By Name(w414) -> ("listbox text"=w412:string[][], "selected values"=w413:i32[])
            n178 = Index Array(array=w413) -> (element=w400:i32)  [unwired: 1 in]
            n179 = Index Array(array=w412, index (row)=w400, index (col)=0 ("disabled index (col)")) -> (element=w409:string)
            n180 = call-poly <vilib>:"NI VeriStand - Set Item Property.vi"("Binary String (T)"=FALSE, "error in (no error)"=w407, "Value"=w409, "Property Name"=w410, "Item Ref in"=w408) -> ("error out"=w406:errorcluster)  [unwired: 4 in, 2 out]
            n181 = control-ref of="Bitfile listbox"() -> (w405:refnum<vi>)
            n182 = call "Bold Row.vi"("error in (no error)"=w406, "Bold? (T)"=FALSE ("Bold?"), "MulticolumnListbox in"=w405) -> ("error out"=w404:errorcluster, "MulticolumnListbox out"=w402:refnum<vi>)  [unwired: 7 in]
            n183 = call "Bold Row.vi"("error in (no error)"=w404, "Row (-2 : all)"=w400, "MulticolumnListbox in"=w402) -> ("error out"=w403:errorcluster)  [unwired: 7 in, 1 out]
          }
          event "Bitfile listbox": Value Change {
            n184 = event-data() -> ("NewVal"=w425:i32[])  [unwired: 1 out]
            n185 = control-ref of="Remove bitfile"() -> (w422:refnum<vi>)
            n186 = control-ref of="Add bitfile"() -> (w423:refnum<vi>)
            n187 = control-ref of="Reload bitfile"() -> (w421:refnum<vi>)
            n188 = control-ref of="Set master"() -> (w420:refnum<vi>)
            n189 = call "Enable Disable Bitfile Buttons.vi"("Set Master in"=w420, "Remove in"=w422, "Reload in"=w421, "Add in"=w423, "error in (no error)"=w426, "NewVal"=w425) -> ("error out"=w424:errorcluster, "NewVal"=w416:i32[])  [unwired: 4 in]
            n190 = Bundle By Name(cluster=w418, "selected values"=w416) -> (w417:T2)
          }
        }
        n191 = call <vilib>:"Simple Error Handler.vi"("error in (no error)"=w92) -> ("error out"=w91:errorcluster)  [unwired: 1 in, 7 out]
        n192 = call <vilib>:"Clear Errors.vi"("error in (no error)"=w91) -> ("error out"=w90:errorcluster)  [unwired: 1 in, 5 out]
      }
      n193 = Unregister For Events(event registration refnum=w84, error in=w83) -> (error out=w82:errorcluster)
    }
    frame Error {
      n194 = call <vilib>:"Simple Error Handler.vi"("error in (no error)"=w429) -> ("error out"=w428:errorcluster)  [unwired: 1 in, 7 out]
      n195 = call <vilib>:"Clear Errors.vi"("error in (no error)"=w428) -> ("error out"=w427:errorcluster)  [unwired: 1 in, 5 out]
    }
  }
  n196 = invoke class="VI" method="FP.Close"(error in=w61) -> (error out=w60:errorcluster)  [unwired: 2 in, 2 out]
  n197 = call <vilib>:"NI VeriStand - Signal When Ready for Shutdown.vi"("error in (no error)"=w60) -> ("error out"=→"error out":errorcluster)  [unwired: 10 out]
